vi "Tilt Calibration (SubVI).vi"(10 "0.1/0.01":bool, 11 "tilt(360)":dbl) -> (3 "tilt":dbl)   [LabVIEW 2018]
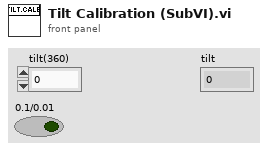
[diagram p1: front panel]
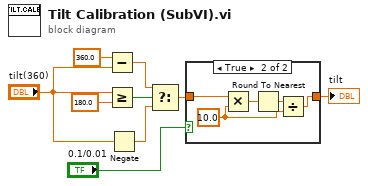
[diagram p0: block diagram]
diagram:
  n1 = Subtract(x=360.0, y="tilt(360)") -> (x-y=w7:dbl)
  n2 = Greater Or Equal?(x="tilt(360)", y=180.0) -> (x >= y?=w5:bool)
  n3 = Negate(x="tilt(360)") -> (-x=w9:dbl)
  n4 = Select(t=w7, s=w5, f=w9) -> (s? t:f=w3:dbl)
  n5 = case shown="True" "0.1/0.01" {
    tunnel: w3 -> [w10 w15]
    tunnel: [w10 w11] -> w2
    frame False {
    }
    frame True {
      w12 = 10.0 ("y")
      n6 = Multiply(x=w15, y=w12) -> (x*y=w14:dbl)
      n7 = Round To Nearest(number=w14) -> (nearest integer value=w13:dbl)
      n8 = Divide(x=w13, y=w12) -> (x/y=w11:dbl)
    }
  }
  "tilt" <- w2
